vi "INIT_Read Test Config File.vi"(8 "error in (no error)":errorcluster) -> (0 "error out 2":errorcluster, 2 "Config\nFile Data":string[][](array[string]))   [LabVIEW 2024]
uses:
  <vilib>/Utility/file.llb/Read Delimited Spreadsheet (string).vi
panel:
  out "size(s)":i32[](array[numeric])
  out "number":u32
  out "Selected File":path
  in  "List of Config CSV files":path[](array[path])=[path "C:/Users/ff107/OneDrive/Documents/GitHub/PWC-OLS/$ConfigFiles/Level Rig ATP OLS-001 Config.csv", path "C:/Users/14407/OneDrive/Allen Aircraft/Level Rig ATP OLS-002 Config.csv"]
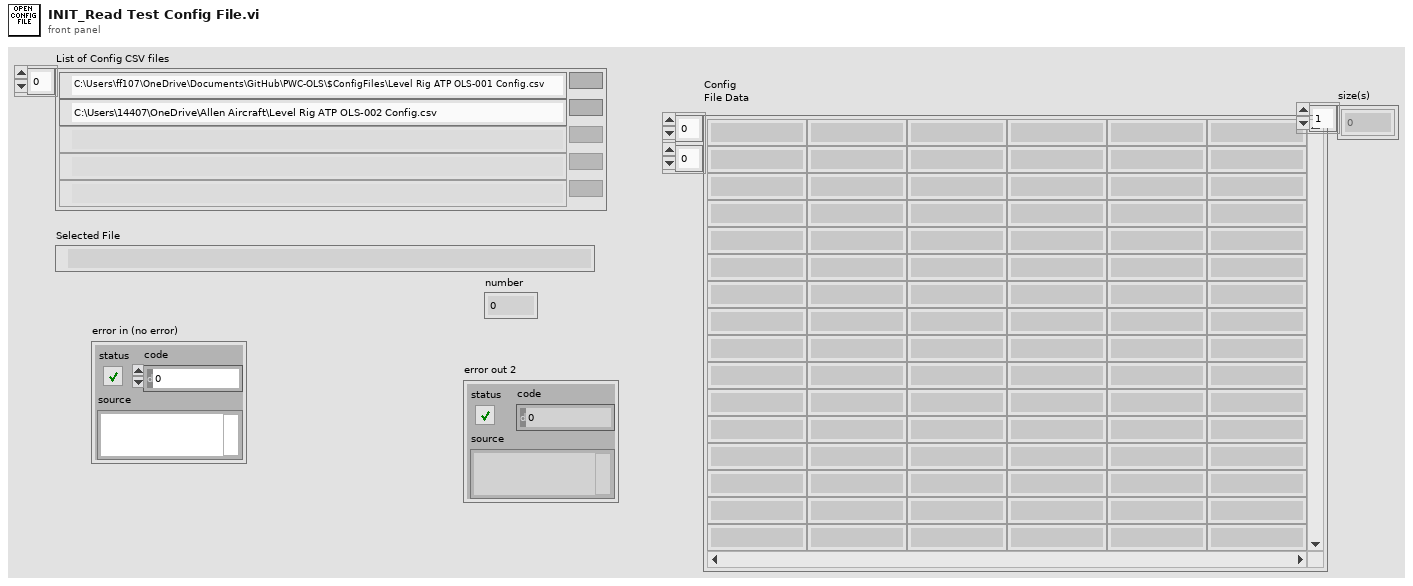
[diagram p1: front panel]
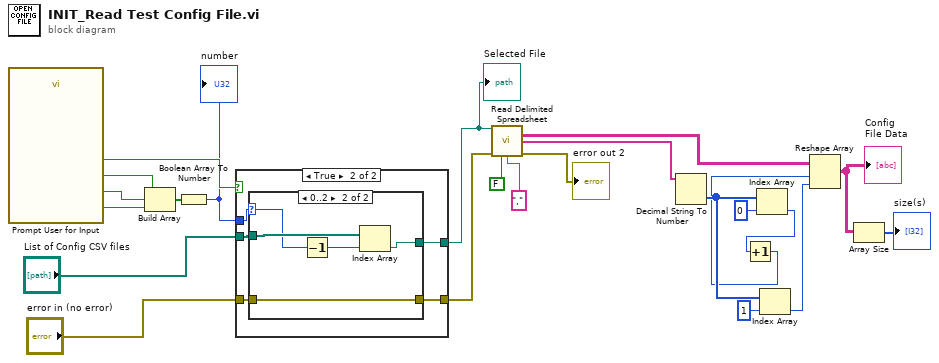
[diagram p0: block diagram]
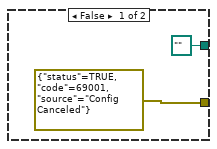
[diagram p2: hidden frame]
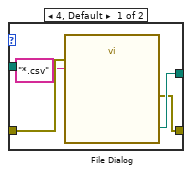
[diagram p3: hidden frame]
diagram:
  n1 = call "Prompt User for Input"() -> ("Browse"=w19:bool, "Oil Level ATP OLS-002"=w20:bool, "Oil Level ATP OLS-001"=w21:bool, "OK"=w17:bool)  [unwired: 15 in, 1 out]
  n2 = Build Array(w21, w20, w19) -> (w18:bool[])
  n3 = Boolean Array To Number(Boolean array=w18) -> (number=w16:u32)
  "number" <- w16
  n4 = case shown="True" w17 {
    tunnel: w16 -> [_ w30]
    tunnel: "List of Config CSV files" -> [_ w29]
    tunnel: "error in (no error)" -> [_ w28]
    tunnel: [errorcluster {"status"=TRUE, "code"=69001, "source"="Config Canceled"} ("error in (no error) 2") w27] -> w13
    tunnel: [path "" ("Path") w26] -> w12
    frame False {
    }
    frame True {
      n5 = case shown="0..2" w30 {
        selector: w30 -> [_ w36]
        tunnel: w29 -> [_ w38]
        tunnel: [w32 w39] -> w27
        tunnel: w28 -> [w33 w39]
        tunnel: [w34 w37] -> w26
        frame 4, Default {
          n6 = call "File Dialog"("error in"=w33, "pattern (all files)"="*.csv") -> ("selected path"=w34:path, "error out"=w32:errorcluster)  [unwired: 10 in, 2 out]
        }
        frame 0..2 {
          n7 = Decrement(x=w36) -> (x-1=w35:u32)
          n8 = Index Array(array=w38, index=w35) -> (element=w37:path)
        }
      }
    }
  }
  "Selected File" <- w12
  n9 = call-poly <vilib>:"Read Delimited Spreadsheet.vi"("file path (dialog if empty)"=w12, "error in (no error)"=w13, "transpose? (F)"=FALSE, "delimiter (\\t)"="," ("delimiter (\\t)")) -> ("all rows"=w9:string[][], "first row"=w10:string[], "error out"=→"error out 2":errorcluster)  [unwired: 6 in, 3 out]
  n10 = Decimal String To Number(string=w10) -> (number=w7:i32[])  [unwired: 2 in, 1 out]
  n11 = Index Array(array=w7, index=0) -> (element=w2:i32)
  n12 = Increment(x=w2) -> (x+1=w1:i32)
  n13 = Index Array(array=w7, index=1) -> (element=w6:i32)
  n14 = Reshape Array(w9, w1, w6) -> (w5:string[][])
  "Config\nFile Data" <- w5
  n15 = Array Size(array=w5) -> (size(s)=→"size(s)":i32[])
